vi "Modbus ComAp Status.vi"(0 "IsGenOn":bool=TRUE, 1 "Alarm":bool=TRUE) -> (5 "Status Out":u16)   [LabVIEW 2014]
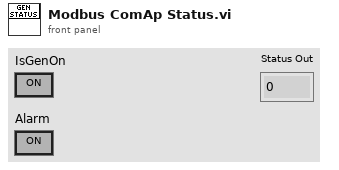
[diagram p1: front panel]
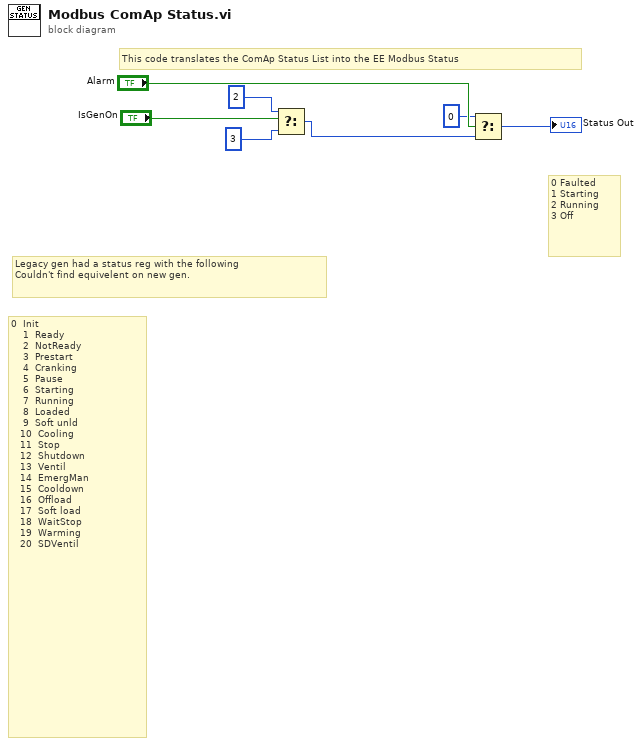
[diagram p0: block diagram]
diagram:
  # "Legacy gen had a status reg with the following\nCouldn't find equivelent on new gen."
  # "0 Faulted\n1 Starting\n2 Running\n3 Off"
  # "0  Init          \n    1  Ready         \n    2  NotReady      \n    3  Prestart      \n    4  Cranking      \n    5  Pause         \n    6  Starting      \n    7  Running       \n    8  Loaded        \n    9  Soft unld     \n   10  Cooling       \n   11  Stop          \n   12  Shutdown      \n   13  Ventil        \n   14  EmergMan      \n   15  Cooldown      \n   16  Offload       \n   17  Soft load     \n   18  WaitStop      \n   19  Warming       \n   20  SDVentil"
  # "This code translates the ComAp Status List into the EE Modbus Status"
  n1 = Select(t=u16 2, s="IsGenOn", f=u16 3) -> (s? t:f=w1:u16)
  n2 = Select(t=u16 0, s="Alarm", f=w1) -> (s? t:f=→"Status Out":u16)
